vi "GUNSC_LibSetArrangeSections_upp.vi"(8 "error in (no error)":errorcluster, 9 "how":string, 11 "Database RefNum out":T1) -> (0 "error out":errorcluster, 1 "response":string, 2 "return value":i32)   [LabVIEW 2016]
uses:
  DBSHAND/private/vis/DatabaseHand_RefNum.ctl
  DBSHAND/private/vis/DatabaseHand_Element_Set(string).vi
  public/c/lib/libunsc.so
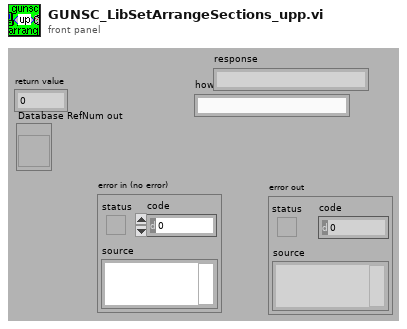
[diagram p1: front panel]
types:
  T1 = typedef "DatabaseHand_RefNum.ctl" = refnum<vi>
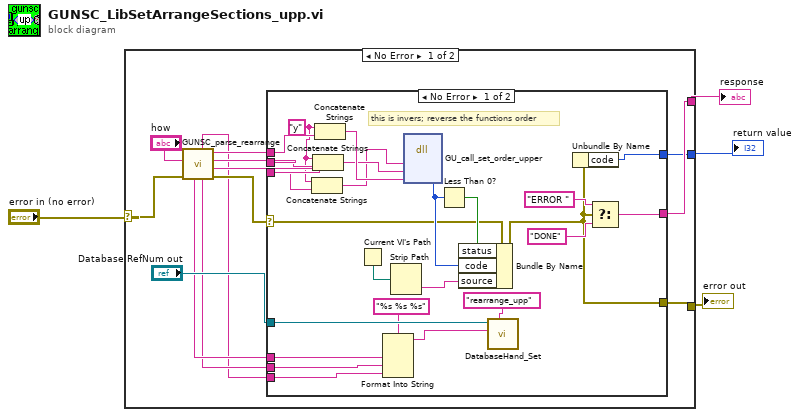
[diagram p0: block diagram]
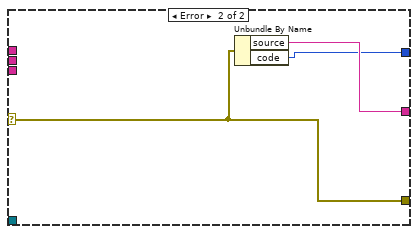
[diagram p2: hidden frame]
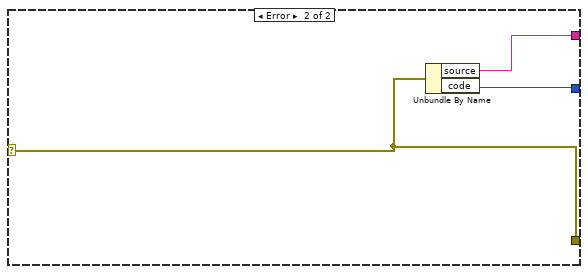
[diagram p3: hidden frame]
diagram:
  n1 = case shown="No Error" "error in (no error)" {
    selector: "error in (no error)" -> [w13 w47]
    tunnel: [w16 w46] -> w4
    tunnel: [w15 w47] -> w2
    tunnel: [w17 w45] -> w1
    frame No Error {
      n2 = call "GUNSC_parse_rearrange.vi"("error in (no error)"=w13, "arguments"="how") -> ("error out"=w12:errorcluster, "func 3"=w9:string, "func 2"=w10:string, "func1"=w11:string, "name2"=w6:string, "name3"=w5:string, "name1"=w7:string)  [unwired: 1 in, 2 out]
      n3 = case shown="No Error" w12 {
        selector: w12 -> [w32 w44]
        tunnel: [w39 w43] -> w17
        tunnel: [w38 w42] -> w16
        tunnel: [w37 w44] -> w15
        tunnel: w11 -> [w24 _]
        tunnel: w10 -> [w22 _]
        tunnel: w9 -> [w19 _]
        tunnel: "Database RefNum out" -> [w31 _]
        tunnel: w7 -> [w27 _]
        tunnel: w6 -> [w26 _]
        tunnel: w5 -> [w25 _]
        frame No Error {
          w20 = "y" ("string")
          # "this is invers; reverse the functions order"
          n4 = Concatenate Strings(w20, w19) -> (w18:string)
          n5 = Concatenate Strings(w20, w22) -> (w21:string)
          n6 = Concatenate Strings(w20, w24) -> (w23:string)
          n7 = Current VI's Path() -> (path=w35:path)
          n8 = Format Into String(format string="%s %s %s", w27, w26, w25) -> (resulting string=w28:string)  [unwired: 2 in, 1 out]
          n9 = Strip Path(path=w35) -> (name=w34:string)  [unwired: 1 out]
          n10 = dll-call lib="home/simager/panview/PAN/Modules/GUNSC/public/c/lib/libunsc.so" fn="GU_call_set_order_upper"("upp1"=w18, "upp2"=w21, "upp3"=w23) -> ("return type"=w36:i32)  [unwired: 6 in, 2 out]
          n11 = Less Than 0?(x=w36) -> (x < 0?=w33:bool)
          n12 = Bundle By Name(cluster=w32, "status"=w33, "code"=w36, "source"=w34) -> (w37:errorcluster)
          n13 = call-poly "DatabaseHand_Set.vi"("name"="rearrange_upp", "value"=w28, "Database RefNum in"=w31) -> ()  [unwired: 5 in, 4 out]
          n14 = Unbundle By Name(w37) -> ("code"=w38:i32)
          n15 = Select(t="ERROR ", s=w37, f="DONE" ("source")) -> (s? t:f=w39:string)
        }
        frame Error {
          n16 = Unbundle By Name(w44) -> ("source"=w43:string, "code"=w42:i32)
        }
      }
    }
    frame Error {
      n17 = Unbundle By Name(w47) -> ("source"=w45:string, "code"=w46:i32)
    }
  }
  "return value" <- w4
  "error out" <- w2
  "response" <- w1
